vi "Unpack Notification Msg.vi"(11 "Notification Msg in":refnum<class "Notification Msg.lvclass">) -> (1 "Publication Time":timestamp, 2 "Value":variant, 3 "Topic Name":string)   [LabVIEW 2015, in "Mediator.lvlib" / "Notification Msg.lvclass"]
uses:
  Notification Msg.lvclass
  Notification Msg.lvclass/Notification Msg.ctl
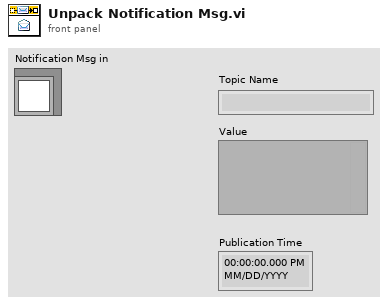
[diagram p1: front panel]
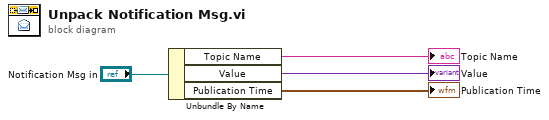
[diagram p0: block diagram]
diagram:
  n1 = Unbundle By Name("Notification Msg in") -> ("Topic Name"=→"Topic Name":string, "Value"=→"Value":variant, "Publication Time"=→"Publication Time":timestamp)
